vi "raster-scanning.vi"() -> ()   [LabVIEW 2015]
uses:
  <vilib>/eio/EIONode/EIONode.xnode
  <vilib>/rvi/eio/common/nirviEmuTemplateMethod_errors.vi
  <vilib>/rvi/DataTransferAndStorage/Container/XNode/niFpgaContainer.xnode
  <vilib>/rvi/DataTransferAndStorage/Register/Emulation/niFpgaRegisterEmulation.vi
  <vilib>/rvi/interface/RandomDataEmulation/nirviRandomDataFpgaReadWriteTemplate.vi
  raster-scan-params.ctl
  controls/boolean_errors.ctl
  controls/PI-params.ctl
panel:
  out "boolean errors":T1
  in  "boolean errors-hidden":T1
  out "ramp-rate":sgl
  in  "x_ffK":sgl
  in  "constant 2 lower":bool
  in  "u(0)":sgl format="%#_13g"
  out "e(0) (threshhold init)":fxp<+/-,16,5>
  out "current-case-selected":i16
  out "trigger":bool
  out "DAC-zaxis":sgl
  out "ADC-zaxis":fxp<+/-,24,5>
  in  "raise-constant":sgl
  in  "initial case":i16=2
  in  "PID to tip up":bool
  in  "raster-scan-params":T2={"TsTicks"=1600, "Stop"=TRUE, "TOL"=0.3, "ramp-rate"=0.0, "z-u-max"=5.0, "PI-params"={"Ki"=0.001, "setpoint"=0.0}} {"z-u-max" format="%#_13g"; "TOL" format="%#_13g"}
  # "DIAGNOSTICS"
  # "TRANSITIONS"
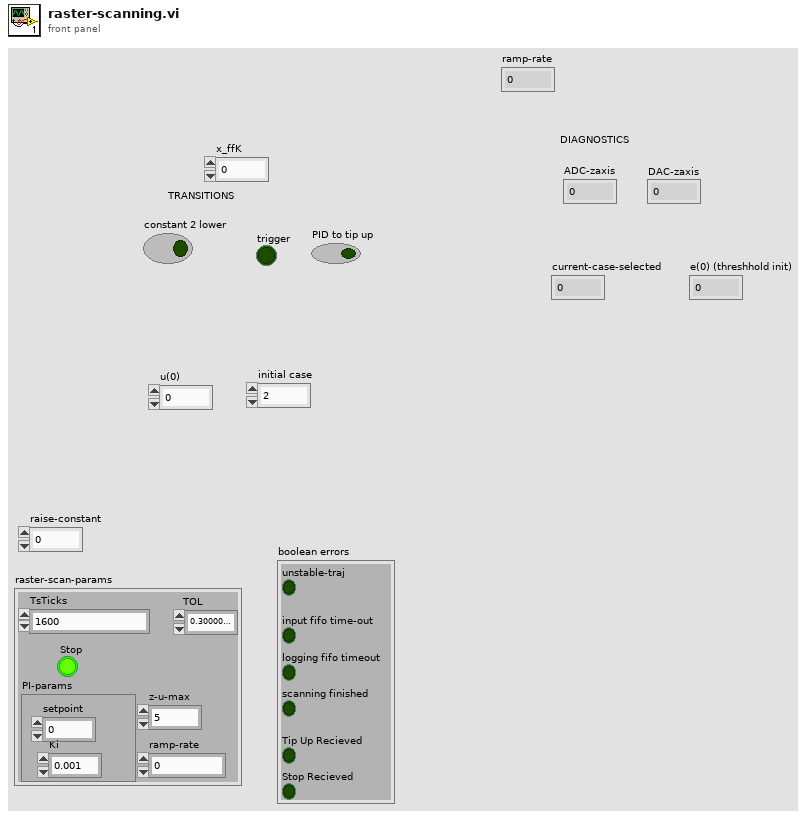
[diagram p1: front panel]
types:
  T1 = typedef "boolean_errors.ctl" = cluster{"unstable-traj":bool, "input fifo time-out":bool, "logging fifo timeout":bool, "scanning finished":bool, "Stop Recieved":bool, "Tip Up Recieved":bool}
  T2 = typedef "raster-scan-params.ctl" = cluster{"TsTicks":u32, "Stop":bool, "TOL":sgl, "ramp-rate":sgl, "z-u-max":sgl, "PI-params":T3}
  T3 = typedef "PI-params.ctl" = cluster{"Ki":sgl, "setpoint":sgl}
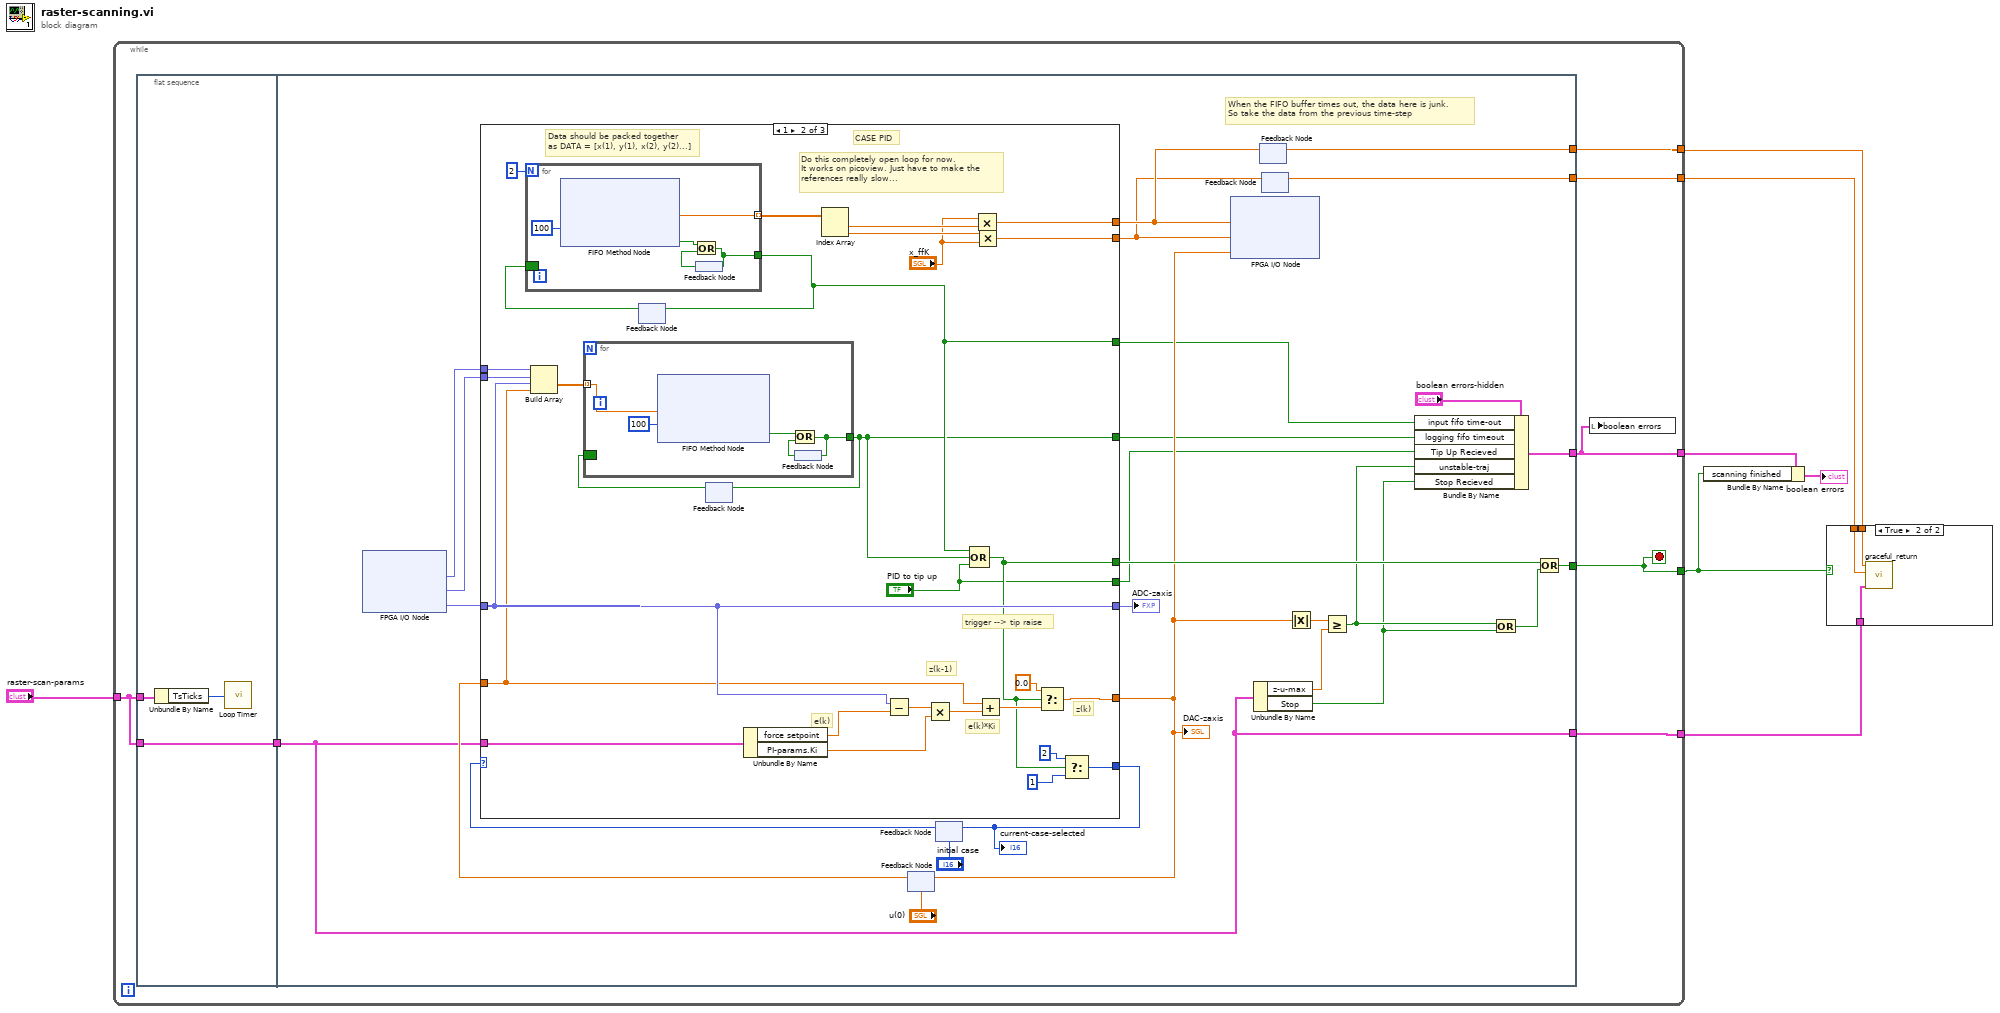
[diagram p0: block diagram]
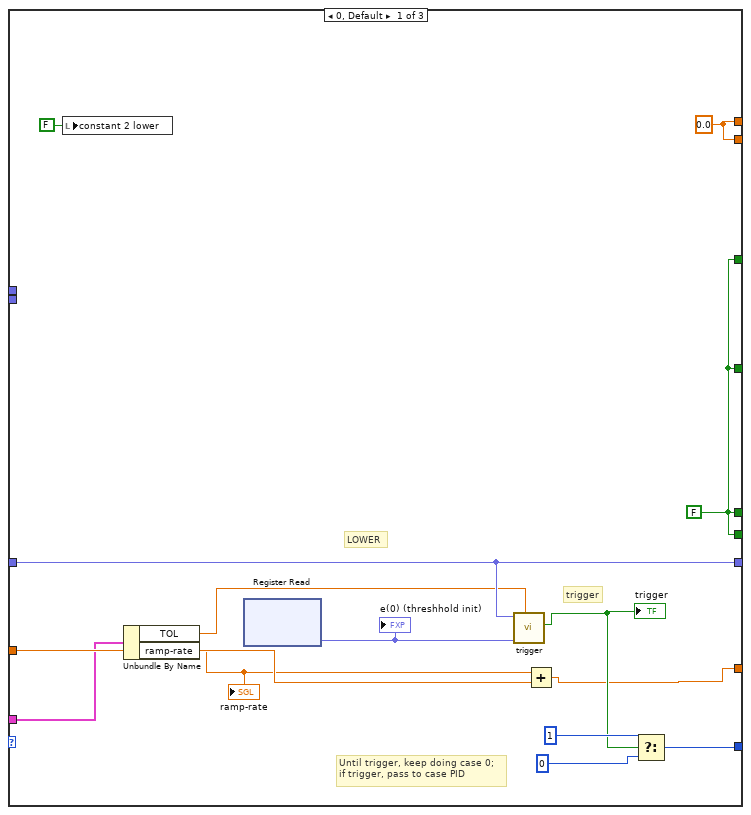
[diagram p3: hidden frame]
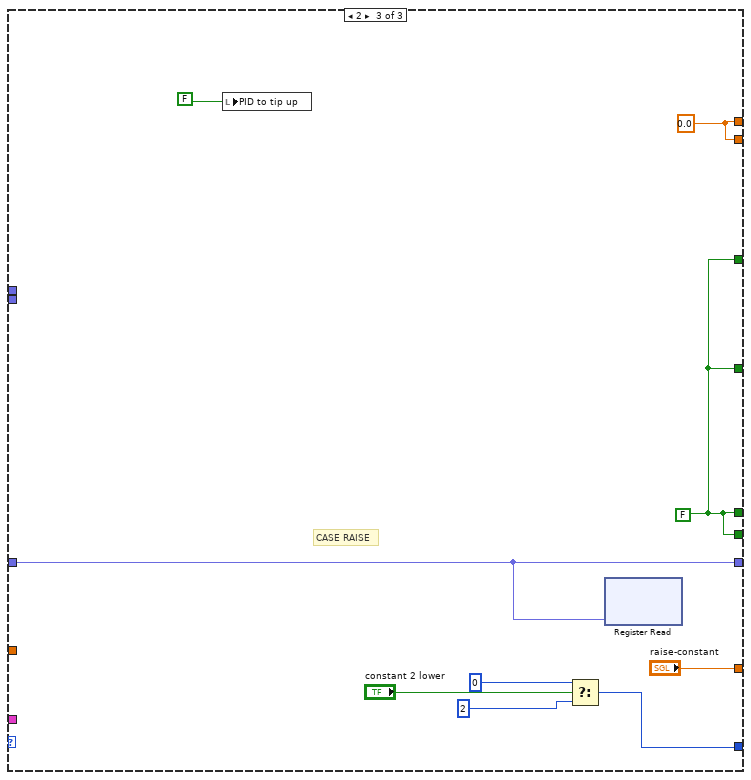
[diagram p4: hidden frame]
diagram:
  n1 = while {
    tunnel: [w14] -> w1
    tunnel: "raster-scan-params" -> [w12]
    tunnel: [w11] -> w4
    tunnel: [w10] -> w6
    tunnel: [w9] -> w5
    tunnel: [w8] -> w3
    stop <- w14 stop-if-true
    n2 = flat-sequence {
      tunnel: w12 -> [w16]
      tunnel: [w15] -> w13
      tunnel: w12 -> [w15]
      tunnel: [w35] -> w14
      tunnel: w13 -> [w29]
      tunnel: [w25] -> w10
      tunnel: [w26] -> w9
      tunnel: [w29] -> w11
      tunnel: [w18] -> w8
      frame #0 {
        n3 = Unbundle By Name(w16) -> ("TsTicks"=w17:u32)
        n4 = call "Loop Timer"("Count(Ticks)"=w17) -> ()  [unwired: 1 out]
      }
      frame #1 {
        # "When the FIFO buffer times out, the data here is junk.\nSo take the data from the previous time-step"
        n5 = xnode "FPGA I/O Node"() -> ("Mod2/AI0"=w37:fxp<+/-,24,5>, "Mod2/AI1"=w38:fxp<+/-,24,5>, "Mod2/AI2"=w44:fxp<+/-,24,5>)  [unwired: 3 in, 3 out]
        n6 = feedback #1("u(0)") -> (w34:sgl)
        n7 = feedback #2("initial case") -> (w39:i16)
        n8 = case shown="1" w39 {
          tunnel: w34 -> [w58 w74 _]
          tunnel: w44 -> [w54 w75 w106]
          tunnel: [w54 w75 w106] -> w43
          tunnel: [w56 w83 w101] -> w41
          tunnel: w38 -> [_ w77 _]
          tunnel: w37 -> [_ w76 _]
          tunnel: [w46 w65 w99] -> w28
          tunnel: [w46 w64 w99] -> w27
          tunnel: [w45 w66 w98] -> w36
          tunnel: [w51 w73 "raise-constant"] -> w32
          tunnel: w29 -> [w49 w72 _]
          tunnel: [w45 w62 w98] -> w23
          tunnel: [w45 w60 w98] -> w22
          tunnel: [w45 "PID to tip up" w98] -> w21
          frame 0, Default {
            w45 = FALSE ("Timed Out?")
            w46 = sgl 0.0 ("Element")
            # "Until trigger, keep doing case 0;\nif trigger, pass to case PID"
            # "LOWER"
            # "trigger"
            n9 = local write "constant 2 lower"(FALSE ("constant 2 lower")) -> ()
            n10 = Unbundle By Name(w49) -> ("TOL"=w48:sgl, "ramp-rate"=w47:sgl)
            "ramp-rate" <- w47
            n11 = xnode ("Register Read")() -> ("Data"=w52:fxp<+/-,16,5>)  [unwired: 1 in, 1 out]
            "e(0) (threshhold init)" <- w52
            n12 = call "trigger.vi"("TOL"=w48, "Vo"=w52, "e(k)"=w54) -> ("trigger"=w53:bool)  [unwired: 8 in]
            "trigger" <- w53
            n13 = Add(x=w47, y=w58) -> (x+y=w51:sgl)
            n14 = Select(t=i16 1, s=w53, f=i16 0) -> (s? t:f=w56:i16)
          }
          frame 1 {
            # "Do this completely open loop for now. \nIt works on picoview. Just have to make the \nreferences really slow..."
            # "Data should be packed together\nas DATA = [x(1), y(1), x(2), y(2)...]"
            # "trigger --> tip raise"
            # "z(k)"
            # "e(k)*Ki"
            # "z(k-1)"
            # "e(k)"
            # "CASE PID"
            n15 = Build Array(w76, w77, w75, w74) -> (w78:sgl[])
            n16 = feedback #3() -> (w63:bool)  [unwired: 1 in]
            n17 = for {
              N: 2 -> [_]
              tunnel: [w97] -> w79 mode=indexing
              tunnel: [w94] -> w62
              border: w63 -> [_]
              n18 = xnode ("FIFO Method Node")("Timeout"=100) -> ("Element"=w97:sgl, "Timed Out?"=w95:bool)  [unwired: 1 in, 1 out]
              n19 = feedback #4() -> (w93:bool)
              n20 = Or(x=w95, y=w93) -> (x .or. y?=w94:bool)
              n21 = feedback-in #4(w94) -> ()
            }
            n22 = feedback-in #3(w62) -> ()
            n23 = feedback #5() -> (w61:bool)  [unwired: 1 in]
            n24 = for {
              tunnel: w78 -> [w92] mode=indexing
              tunnel: [w88] -> w60
              border: w61 -> [_]
              n25 = xnode ("FIFO Method Node")("Element"=w92, "Timeout"=100) -> ("Timed Out?"=w90:bool)  [unwired: 1 in, 1 out]
              n26 = feedback #6() -> (w89:bool)
              n27 = Or(x=w90, y=w89) -> (x .or. y?=w88:bool)
              n28 = feedback-in #6(w88) -> ()
            }
            n29 = feedback-in #5(w60) -> ()
            n30 = Unbundle By Name(w72) -> ("force setpoint"=w71:sgl, "PI-params.Ki"=w70:sgl)
            n31 = Index Array(array=w79) -> (element #1=w69:sgl, element #2=w68:sgl)  [unwired: 2 in]
            n32 = Subtract(x=w75, y=w71) -> (x-y=w87:sgl)
            n33 = Multiply(x=w87, y=w70) -> (x*y=w86:sgl)
            n34 = Compound Arithmetic op=OR(w62, w60, "PID to tip up") -> (w66:bool)
            n35 = Multiply(x="x_ffK", y=w69) -> (x*y=w65:sgl)
            n36 = Multiply(x=w68, y="x_ffK") -> (x*y=w64:sgl)
            n37 = Add(x=w74, y=w86) -> (x+y=w85:sgl)
            n38 = Select(t=sgl 0.0 ("f"), s=w66, f=w85) -> (s? t:f=w73:sgl)
            n39 = Select(t=i16 2, s=w66, f=i16 1) -> (s? t:f=w83:i16)
          }
          frame 2 {
            w98 = FALSE ("Timed Out?")
            w99 = sgl 0.0 ("Element")
            # "CASE RAISE"
            n40 = local write "PID to tip up"(FALSE) -> ()
            n41 = Select(t=i16 0 ("f"), s="constant 2 lower", f=i16 2) -> (s? t:f=w101:i16)
            n42 = xnode ("Register Read")("Data"=w106) -> ()  [unwired: 1 in, 1 out]
          }
        }
        "ADC-zaxis" <- w43
        "DAC-zaxis" <- w32
        "current-case-selected" <- w41
        n43 = feedback-in #1(w32) -> ()
        n44 = feedback-in #2(w41) -> ()
        n45 = xnode "FPGA I/O Node"("Mod1/AO0"=w28, "Mod1/AO1"=w27, "Mod1/AO2"=w32) -> ()  [unwired: 3 in, 3 out]
        n46 = Unbundle By Name(w29) -> ("z-u-max"=w31:sgl, "Stop"=w19:bool)
        n47 = feedback-in #7(w28) -> ()
        n48 = feedback #7() -> (w25:sgl)  [unwired: 1 in]
        n49 = feedback #8() -> (w26:sgl)  [unwired: 1 in]
        n50 = feedback-in #8(w27) -> ()
        n51 = Absolute Value(x=w32) -> (abs(x)=w42:sgl)
        n52 = Greater Or Equal?(x=w42, y=w31) -> (x >= y?=w20:bool)
        n53 = Bundle By Name(cluster="boolean errors-hidden", "input fifo time-out"=w23, "logging fifo timeout"=w22, "Tip Up Recieved"=w21, "unstable-traj"=w20, "Stop Recieved"=w19) -> (w18:T1)
        n54 = Or(x=w20, y=w19) -> (x .or. y?=w30:bool)
        n55 = Or(x=w36, y=w30) -> (x .or. y?=w35:bool)
      }
    }
    n56 = local write "boolean errors"(w8) -> ()
  }
  n57 = Bundle By Name(cluster=w3, "scanning finished"=w1) -> (→"boolean errors":T1)
  n58 = case shown="True" w1 {
    tunnel: w6 -> [_ w109]
    tunnel: w5 -> [_ w108]
    tunnel: w4 -> [_ w107]
    frame False {
    }
    frame True {
      n59 = call "graceful_return.vi"("raster-scan-params"=w107, "uy(0)"=w108, "ux(0)"=w109) -> ()  [unwired: 9 in]
    }
  }
